vi "Untitled 1.vi"(6 "Device Class":string="FakeCamSub", 7 "index of element 2":i32, 8 "data":string[][](array[string]), 9 "index of element":i32) -> (0 "All Devices":string[](array[string]), 1 "data 2":string[][](array[string]), 2 "index (row)":i32, 3 "String":string)   [LabVIEW 2013]
uses:
  shared programs/MySQL/Preset Query Enum.ctl
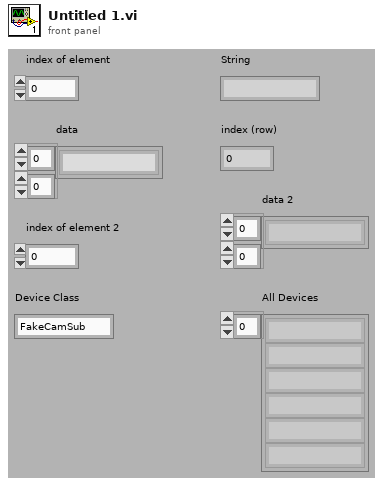
[diagram p1: front panel]
types:
  T1 = typedef "Preset Query Enum.ctl" = enum16{"Get Locations", "Get all IPs and MACs", "Get classes", "Get expt variables to set at scanstart for particular device", "Get expt devices and variables with start values", "Get expt devices and variables (with data to get)", "Get expt devices with data to get", "Get Expt devices and GUIs", "Get all devices basic properties", "Get Virtual Devices Core Info", "Get Expt names", "Get experiment basic properties", "Get experiment alarm variables", "Get MC Ports", "Get device network comm port", "Get devicetype lvclass path", "Get basic device properties", "Get Init Order", "Get all setable variables of a device", "Get device variable aliases", "Get force values of all settable variables", "Get all variables of a devicetype", "Get all variables of a device", "Get plotter details", "Get Saved Scans", "Get Scan Info", "GetGeneralGUIs", "Get expt for plotter", "Get plotter IDs from expt", "Get all devices", "Get all Virtual Devices", "Get variable and device info for Virtual Device", "GetItemLocatorIP", "Get IPs for GUIs", "Get DeviceType from Device", "GetLocalPortRange", "GetDevicePresetVariables", "Get Device Configuration", "GetAllPresetNames", "GetAllConfigurationNames", "GetPresetDeviceNames"}
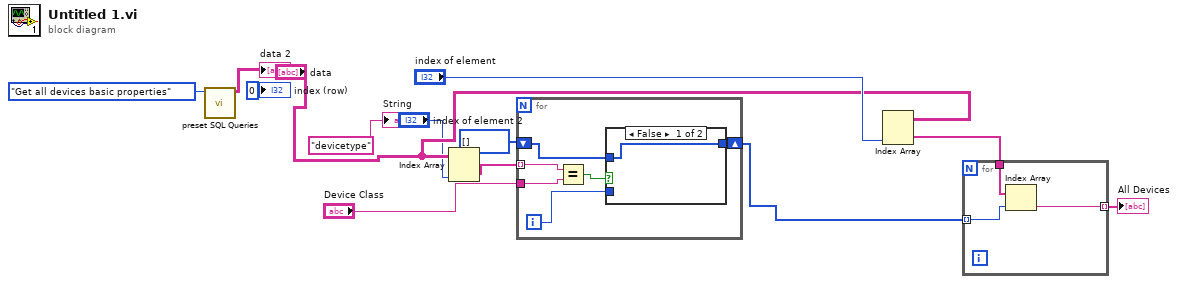
[diagram p0: block diagram]
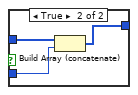
[diagram p2: hidden frame]
diagram:
  n1 = call "preset SQL Queries.vi"("Preset Query"=Preset_Query_Enum."Get all devices basic properties") -> ("data"=→"data 2":string[][])  [unwired: 8 in, 2 out]
  n2 = Index Array(array="data", index (col)="index of element 2") -> (element=w6:string[])  [unwired: 1 in]
  n3 = for {
    tunnel: w6 -> [w19] mode=indexing
    tunnel: "Device Class" -> [w18]
    shift-right: [w15] -> w11
    shift-left: i32[] [] -> [w14]
    i -> [w16]
    n4 = Equal?(x=w19, y=w18) -> (x = y?=w17:bool)
    n5 = case shown="False" w17 {
      tunnel: w16 -> [_ w23]
      tunnel: [w20 w22] -> w15
      tunnel: w14 -> [w20 w21]
      frame False {
      }
      frame True {
        n6 = Build Array (concatenate)(w21, w23) -> (w22:i32[])
      }
    }
  }
  n7 = Index Array(array="data", index (col)="index of element") -> (element=w12:string[])  [unwired: 1 in]
  n8 = for {
    tunnel: w11 -> [w25] mode=indexing
    tunnel: w12 -> [w26]
    tunnel: [w24] -> w13 mode=indexing
    n9 = Index Array(array=w26, index=w25) -> (element=w24:string)
  }
  "All Devices" <- w13
  "index (row)" <- 0 ("index (row)")
  "String" <- "devicetype"
